vi "CAL-Plot data.vi"(0 "Path":path, 1 "Name":string, 5 "Mag graph":refnum<vi>, 7 "Phase graph":refnum<vi>, 9 "Plot.Line Width":u8=2, 11 "error in (no error)":errorcluster, 12 "Plot Max SPL (F)":bool) -> (4 "Path (out)":path, 15 "error out":errorcluster)   [LabVIEW 2020]
doc: "This helper VI loads calibration data from a file, and plots the magnitude and phase on graphs whose references are inputs to the VI. Handles the logic of overplotting data, selecting the colors and linestyles, and inserting the filename into the legend.\n\nKEH 9/10/09"
uses:
  PXI DAQ VIs/DAQ Engine VIs/PXI Globals.vi
  Utility VIs/Math VIs/Linear to dB (scalar).vi
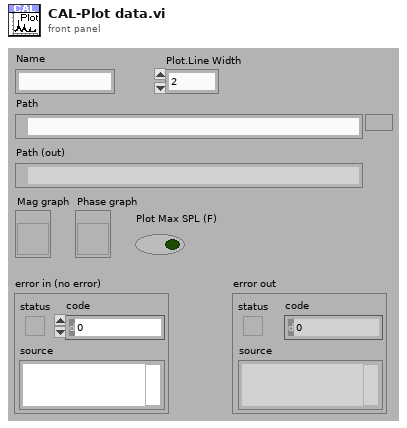
[diagram p1: front panel]
types:
  T1 = cluster{"Frequency (Hz)":dbl[], "PTC Phase":dbl[]}[]
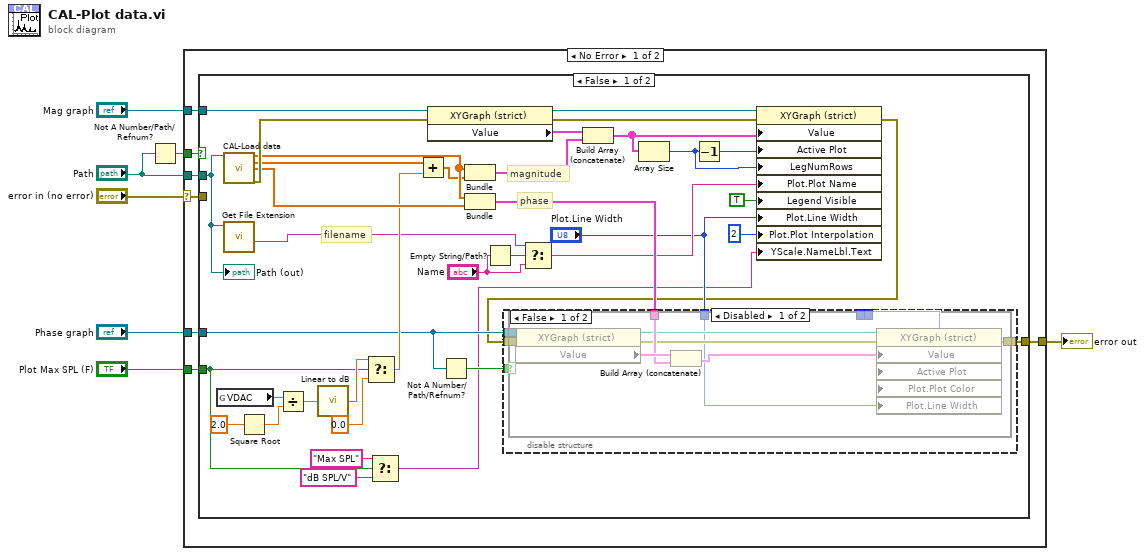
[diagram p0: block diagram]
diagram:
  n1 = Not A Number/Path/Refnum?(number/path/refnum="Path") -> (NaN/Path/Refnum?=w4:bool)
  n2 = case shown="No Error" "error in (no error)" {
    selector: "error in (no error)" -> [w9 w73]
    tunnel: "Mag graph" -> [w14 _]
    tunnel: "Phase graph" -> [w13 _]
    tunnel: [w12 w73] -> w5
    tunnel: w4 -> [w11 _]
    tunnel: "Path" -> [w10 _]
    tunnel: "Plot Max SPL (F)" -> [w8 _]
    frame No Error {
      n3 = case shown="False" w11 {
        tunnel: w14 -> [w51 _]
        tunnel: w9 -> [_ w72]
        tunnel: w13 -> [w29 _]
        tunnel: [w47 w72] -> w12
        tunnel: w10 -> [w16 _]
        tunnel: w8 -> [w34 _]
        frame False {
          # "filename"
          # "phase"
          # "magnitude"
          n4 = global read "PXI Globals.vi" "VDAC"() -> (w37:dbl)
          n5 = call "CAL-Load data.vi"("user path"=w16) -> ("Frequency (Hz)"=w45:dbl[], "Mag"=w43:dbl[], "Phase"=w44:dbl[], "error out"=w50:errorcluster)  [unwired: 7 in, 4 out]
          n6 = call <vilib>:"Get File Extension.vi"("file"=w16) -> ("filename without extension"=w15:string)  [unwired: 6 in, 4 out]
          n7 = Square Root(x=2.0) -> (sqrt(x)=w38:dbl)
          n8 = Divide(x=w37, y=w38) -> (x/y=w40:dbl)
          n9 = call-poly "Linear to dB.vi"("Linear"=w40) -> ("dB"=w35:dbl)
          n10 = Select(t=w35, s=w34, f=0.0) -> (s? t:f=w36:dbl)
          n11 = Select(t="Max SPL", s=w34, f="dB SPL/V") -> (s? t:f=w18:string)
          n12 = Add(x=w43, y=w36) -> (x+y=w42:dbl[])
          n13 = property class="XYGraph (strict)"(reference=w51, error in=w50) -> (reference out=w27:refnum<vi>, error out=w26:errorcluster, "Value"=w49:cluster{"PTC Mag":dbl[], "PTC Phase":dbl[]}[])
          n14 = Not A Number/Path/Refnum?(number/path/refnum=w29) -> (NaN/Path/Refnum?=w28:bool)
          n15 = Bundle("Frequency (Hz)"=w45, w42) -> (w46:cluster{"Frequency (Hz)":dbl[], dbl[]})  [unwired: 1 in]
          n16 = Bundle("Frequency (Hz)"=w45, "Phase"=w44) -> (w48:cluster{"Frequency (Hz)":dbl[], "Phase":dbl[]})  [unwired: 1 in]
          n17 = Empty String/Path?(string/path="Name") -> (empty?=w31:bool)
          n18 = Select(t=w15, s=w31, f="Name") -> (s? t:f=w22:string)
          n19 = Build Array (concatenate)(w49, w46) -> (w25:T1)
          n20 = Array Size(array=w25) -> (size(s)=w23:i32)
          n21 = Decrement(x=w23) -> (x-1=w24:i32)
          n22 = property class="XYGraph (strict)"(reference=w27, error in=w26, "Value"=w25, "Active Plot"=w24, "LegNumRows"=w23, "Plot.Plot Name"=w22, "Legend Visible"=TRUE ("Legend:Visible"), "Plot.Line Width"="Plot.Line Width", "Plot.Plot Interpolation"=u8 2, "YScale.NameLbl.Text"=w18) -> (error out=w17:errorcluster)  [unwired: 1 out]
          n23 = disable-structure shown="Disabled" {
            disable-tunnel: w17 -> [w59 _]
            disable-tunnel: w48 -> [w58 _]
            disable-tunnel: [w57 _] -> w47
            disable-tunnel: _ -> [w56 _]
            disable-tunnel: _ -> [w55 _]
            disable-tunnel: "Plot.Line Width" -> [w54 _]
            disable-tunnel: w29 -> [w53 _]
            disable-tunnel: w28 -> [w52 _]
            frame Disabled {
              n24 = case shown="False" w52 {
                tunnel: w53 -> [w70 _]
                tunnel: w59 -> [w69 w71]
                tunnel: w58 -> [w67 _]
                tunnel: [w63 w71] -> w57
                tunnel: w56 -> [w62 _]
                tunnel: w55 -> [w61 _]
                tunnel: w54 -> [w60 _]
                frame False {
                  n25 = property class="XYGraph (strict)"(reference=w70, error in=w69) -> (reference out=w66:refnum<vi>, error out=w65:errorcluster, "Value"=w68:cluster{"PTC Mag":dbl[], "PTC Phase":dbl[]}[])
                  n26 = Build Array (concatenate)(w68, w67) -> (w64:cluster{"Frequency (Hz)":dbl[], "Phase":dbl[]}[])
                  n27 = property class="XYGraph (strict)"(reference=w66, error in=w65, "Value"=w64, "Active Plot"=w62, "Plot.Plot Color"=w61, "Plot.Line Width"=w60) -> (error out=w63:errorcluster)  [unwired: 1 out]
                }
                frame True {
                }
              }
            }
            frame Enabled {
            }
          }
          "Path (out)" <- w16
        }
        frame True {
        }
      }
    }
    frame Error {
    }
  }
  "error out" <- w5
